vi "DrumSequence_Cont_Execute.vi"(4 "Set Next Step":bool, 6 "Pass_Through_Time":dbl=-1.0 format="%33.4f", 7 "External Ready":bool=TRUE, 8 "Cancel Time Sec":dbl, 9 "Step Times Sec":dbl[](array[numeric]), 10 "Cancel":bool, 11 "Initiate":bool) -> (0 "Error":bool, 1 "Ready":bool, 2 "Seq  Active":bool, 3 "Step Number State":T1=enum."Initialize", 5 "New Step":bool)   [LabVIEW 2019, in "Trajectory_Library.lvlib"]
doc: "Implements a simplified state machine similar to a mechanical / electrical drum sequencer. When the Drum Sequencer is \"Ready\" and the \"Initiate\" input becomes TRUE,, the drum sequences through its set of steps from 1 to N. After each Step is executed it is followed by a wait. During the wait the Step output indicates \"Do Nothing\". The number of Steps is determined by the number of elements in the \"Step Times\" input array. Once all the steps have been executed, the Drum Sequencer cycles bac to wait for another initiate. \n\nThere is a Cancel input that interrupts the sequence, executes the Cancel Step, performs the cancel wait, and then returns to wait for an Initiate action. \n\nIf any of the Step Times, or Cancel times are negative, or there more than 32 steps, or less than 1 step an error is signaled. The drum sequencer selects the error state and stays there.\n\nInputs:\n\nOutputs:"
uses:
  Trajectory_Library.lvlib
  Enum/DrumSequence_Step_Enum.ctl
  Enum/DrumSequence_State_Enum.ctl
  Util_GetTime_U32.vi
  Util_GetTime_U64.vi
  <vilib>/Utility/semaphor.llb/Obtain Semaphore Reference.vi
  Timer_Reset.vi
panel:
  # "Time to wait\nafter executing\nstep"
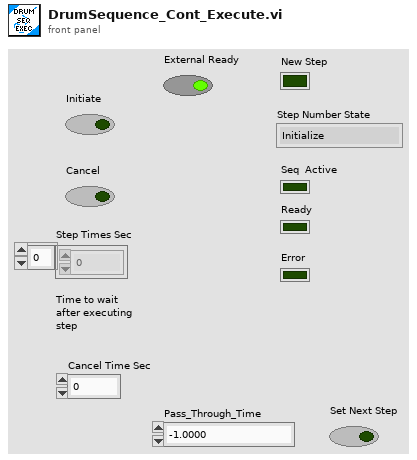
[diagram p1: front panel]
types:
  T1 = typedef "Trajectory_Library.lvlib/DrumSequence_Step_Enum.ctl" = enum16{"Do Nothing", "Step 1", "Step 2", "Step 3", "Step 4", "Step 5", "Step 6", "Step 7", "Step 8", "Step 9", "Step 10", "Step 11", "Step 12", "Step 13", "Step 14", "Step 15", "Step 16", "Step 17", "Step 18", "Step 19", "Step 20", "Step 21", "Step 22", "Step 23", "Step 24", "Step 25", "Step 26", "Step 27", "Step 28", "Step 29", "Step 30", "Step 31", "Step 32", "Cancel", "Initialize", "Error"}
  T2 = typedef "Trajectory_Library.lvlib/DrumSequence_State_Enum.ctl" = enum16{"Initialize", "Ready", "First Step", "Step Wait", "Next State", "Cancel", "Cancel Wait", "Error", "Error Loop"}
  T3 = typedef "Trajectory_Library.lvlib/TIMER.ctl" = cluster{"StartTime":dbl, "Accumulated TIme":dbl, "Running":bool, "semaphore":T4}
  T4 = typedef "Semaphore RefNum" = refnum<k1>
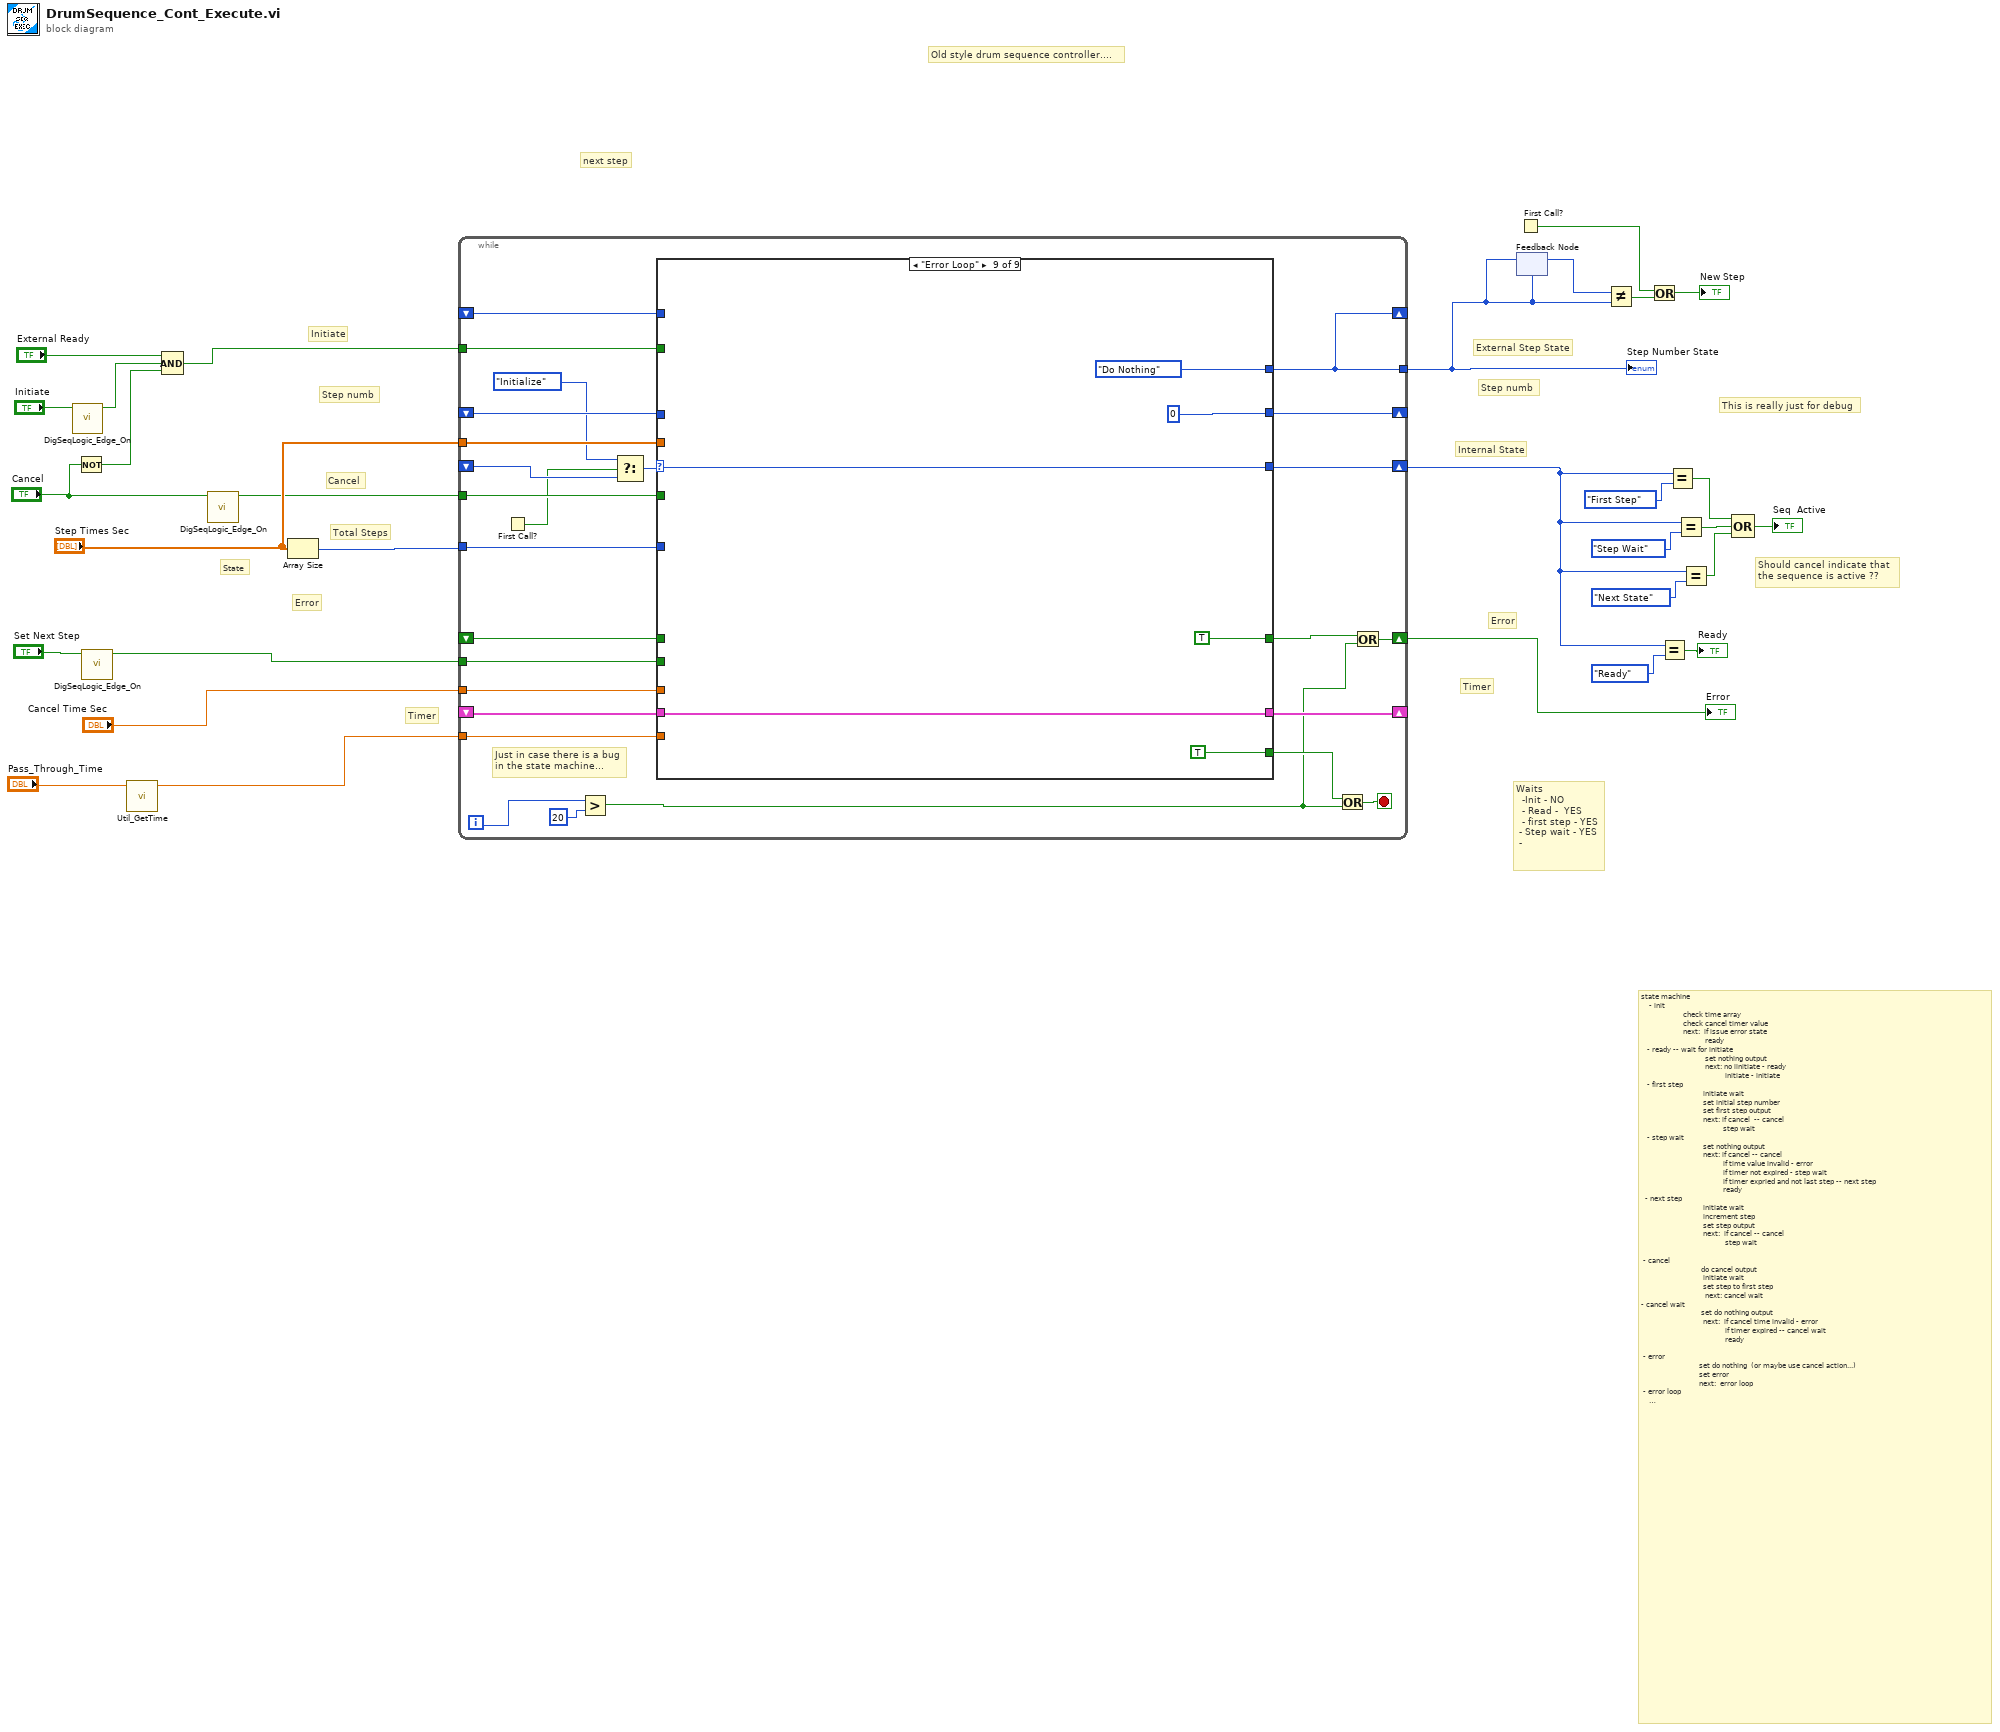
[diagram p0: block diagram]
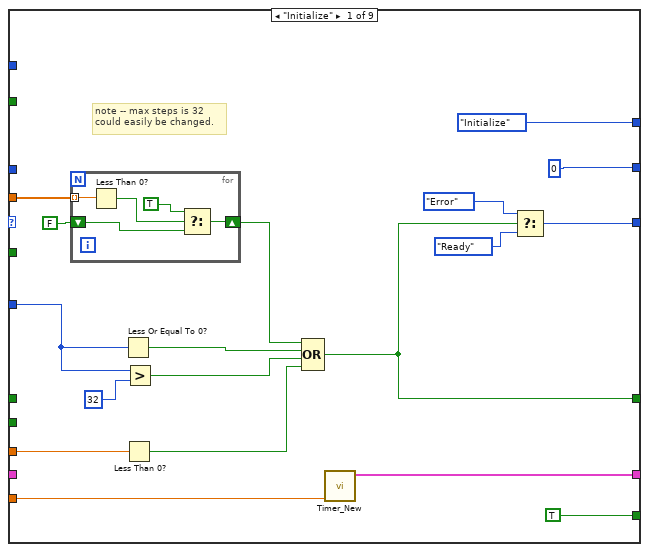
[diagram p2: hidden frame]
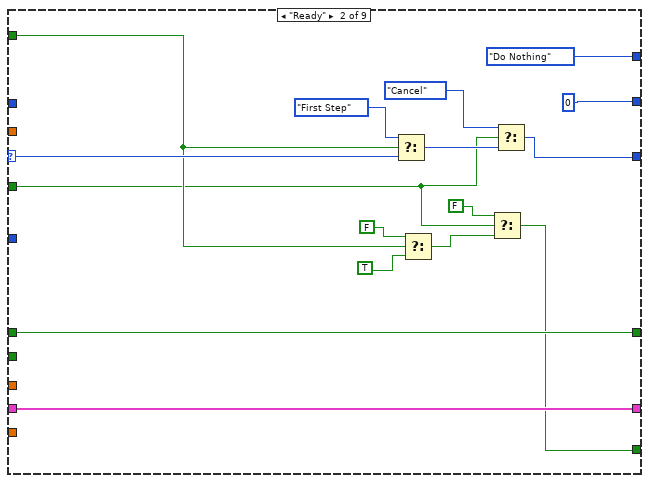
[diagram p3: hidden frame]
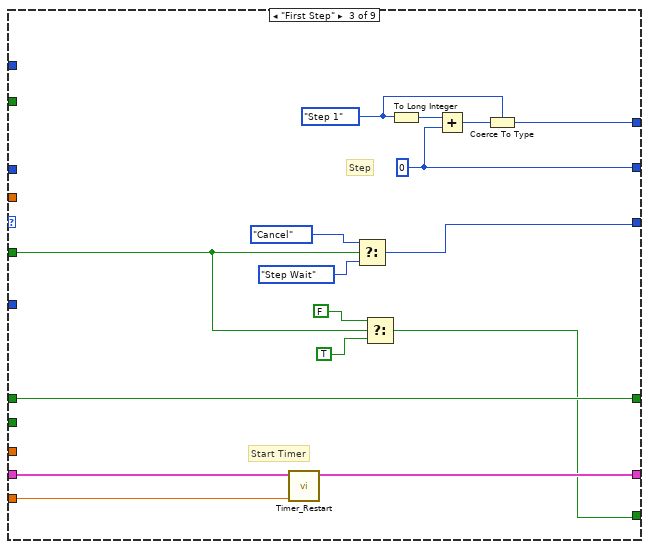
[diagram p4: hidden frame]
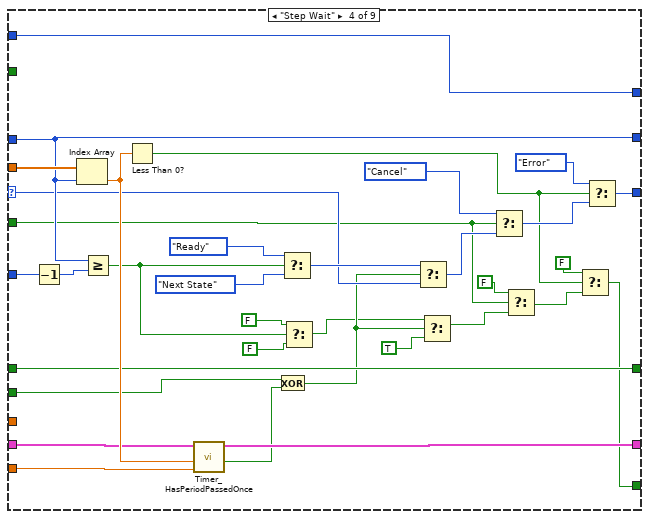
[diagram p5: hidden frame]
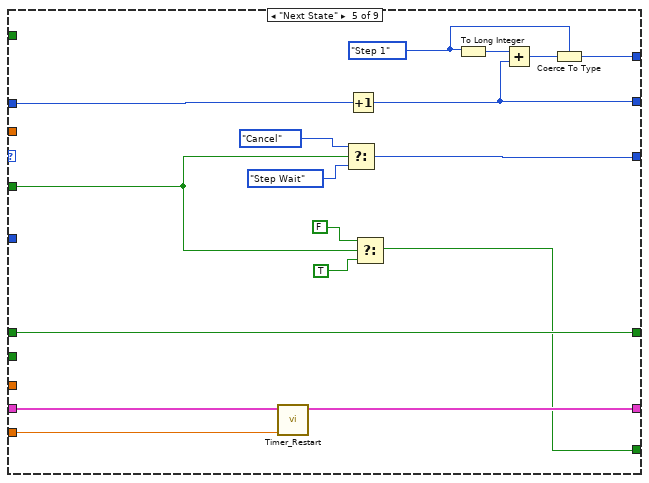
[diagram p6: hidden frame]
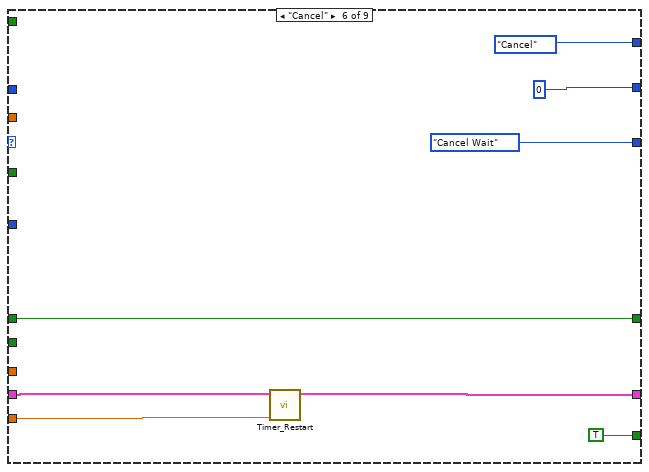
[diagram p7: hidden frame]
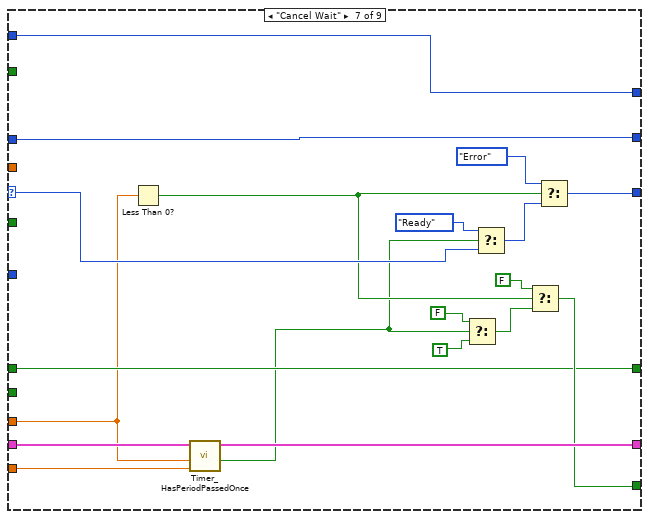
[diagram p8: hidden frame]
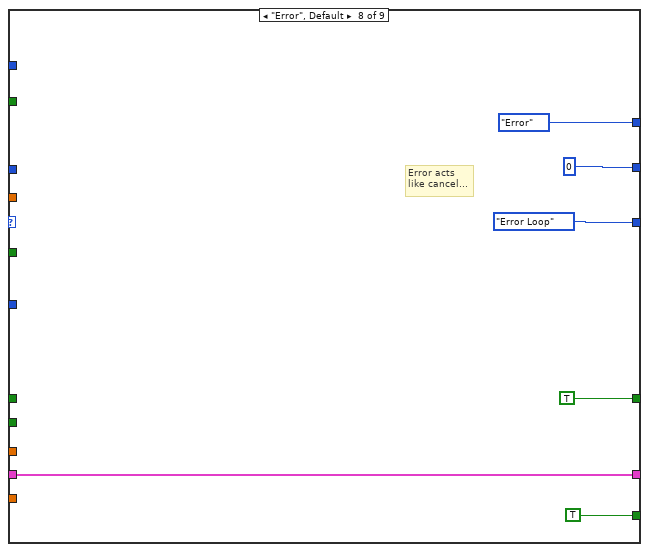
[diagram p9: hidden frame]
diagram:
  # "Should cancel indicate that\nthe sequence is active ??"
  # "This is really just for debug"
  # "Waits\n  -Init - NO\n  - Read -  YES\n  - first step - YES\n - Step wait - YES\n -"
  # "Timer"
  # "Error"
  # "State"
  # "Total Steps"
  # "Cancel"
  # "Step numb"
  # "Initiate"
  # "next step"
  # "Old style drum sequence controller...."
  # "Step numb"
  # "Timer"
  # "Error"
  # "Internal State"
  # "External Step State"
  # "state machine\n    - init\n                     check time array\n                     check cancel timer value\n                     next:  if issue error state\n                                ready\n   - ready -- wait for initiate\n                                set nothing output\n                                next: no iinitiate - ready\n                                          initiate - initiate\n   - first step \n                               initiate wait\n                               set initial step number\n                               set first step output\n                               next: if cancel  -- cancel\n                                         step wait\n   - step wait \n                               set nothing output\n                               next: if cancel -- cancel\n                                         if time value invalid - error\n                                         if timer not expired - step wait\n                                         if timer expried and not last step -- next step\n                                         ready\n  - next step\n                               initiate wait\n                               increment step\n                               set step output\n                               next:  if cancel -- cancel\n                                          step wait\n\n - cancel\n                              do cancel output\n                               initiate wait\n                               set step to first step\n                                next: cancel wait\n- cancel wait\n                              set do nothing output\n                               next:  if cancel time invalid - error\n                                          if timer expired -- cancel wait\n                                          ready\n\n - error\n                             set do nothing  (or maybe use cancel action...)\n                             set error\n                             next:  error loop\n - error loop\n                             set do nothing\n                             set error\n                             next: error loop"
  n1 = call "DigSeqLogic_Edge_On.vi"("Input"="Initiate") -> ("On Edge"=w28:bool)  [unwired: 10 in]
  n2 = Not(x="Cancel") -> (.not. x?=w30:bool)
  n3 = call "DigSeqLogic_Edge_On.vi"("Input"="Set Next Step") -> ("On Edge"=w9:bool)  [unwired: 10 in]
  n4 = call "Util_GetTime.vi"("Pass_Through_Time"="Pass_Through_Time") -> ("FPGA_Time_Seconds"=w23:dbl)  [unwired: 8 in, 2 out]
  n5 = Compound Arithmetic op=AND("External Ready", w28, w30) -> (w22:bool)
  n6 = call "DigSeqLogic_Edge_On.vi"("Input"="Cancel") -> ("On Edge"=w6:bool)  [unwired: 10 in]
  n7 = Array Size(array="Step Times Sec") -> (size(s)=w27:i32)
  n8 = while {
    tunnel: "Step Times Sec" -> [w55]
    tunnel: "Cancel Time Sec" -> [w54]
    tunnel: w23 -> [w53]
    tunnel: w22 -> [w52]
    tunnel: w6 -> [w51]
    tunnel: [w32] -> w1
    tunnel: w9 -> [w48]
    tunnel: w27 -> [w56]
    shift-right: [w47] -> _
    shift-left: _ -> [w41]
    shift-right: [w35] -> w8
    shift-left: _ -> [w46]
    shift-right: [w49] -> w12
    shift-left: _ -> [w43]
    shift-right: [w50] -> _
    shift-left: _ -> [w45]
    shift-right: [w32] -> _
    shift-left: _ -> [w31]
    i -> [w37]
    stop <- w39 stop-if-true
    # "Just in case there is a bug\nin the state machine..."
    n9 = First Call?() -> (First Call?: T/F=w40:bool)
    n10 = Greater?(x=w37, y=20) -> (0:w33:bool)
    n11 = Select(t=DrumSequence_State_Enum."Initialize", s=w40, f=w43) -> (s? t:f=w44:T2)
    n12 = case shown="\"Error Loop\"" w44 {
      selector: w44 -> [_ w94 _ w132 _ _ w183 _ w200]
      tunnel: w56 -> [w63 _ _ w130 _ _ _ _ _]
      tunnel: w55 -> [w73 _ _ w138 _ _ _ _ _]
      tunnel: w54 -> [w72 _ _ _ _ _ w173 _ _]
      tunnel: [w69 w91 w101 w126 w148 w165 w176 TRUE TRUE] -> w34
      tunnel: [w66 w84 w96 w135 w155 DrumSequence_State_Enum."Cancel Wait" w186 DrumSequence_State_Enum."Error Loop" w200] -> w49
      tunnel: [w65 w90 w106 w144 w153 w168 w187 w190 w197] -> w47
      tunnel: w53 -> [w64 _ w107 w145 w154 w169 w175 _ _]
      tunnel: [DrumSequence_Step_Enum."Initialize" ("Step Number") DrumSequence_Step_Enum."Do Nothing" ("Step Number") w109 w112 w156 DrumSequence_Step_Enum."Cancel" ("Step Number") w171 DrumSequence_Step_Enum."Error" ("Step Number") DrumSequence_Step_Enum."Do Nothing" ("Step Number")] -> w32
      tunnel: w52 -> [_ w89 _ _ _ _ _ _ _]
      tunnel: [0 0 w108 w133 w157 0 w184 0 0] -> w50
      tunnel: w51 -> [_ w81 w100 w118 w149 _ _ _ _]
      tunnel: w45 -> [_ _ _ w133 w158 _ w184 _ _]
      tunnel: w48 -> [_ _ _ w128 _ _ _ _ _]
      tunnel: w41 -> [_ w90 w102 w127 w147 w163 w174 w190 w197]
      tunnel: w46 -> [_ w91 w101 w126 w148 w165 w176 _ _]
      tunnel: [TRUE w80 w97 w113 w146 TRUE w178 TRUE TRUE] -> w38
      tunnel: w31 -> [_ _ _ w112 _ _ w171 _ _]
      frame "Initialize" {
        # "note -- max steps is 32\ncould easily be changed."
        n13 = for {
          shift-right: [w78] -> w71
          shift-left: FALSE -> [w77]
          tunnel: w73 -> [w79] mode=indexing
          n14 = Less Than 0?(x=w79) -> (x < 0?=w75:bool)
          n15 = Select(t=TRUE, s=w75, f=w77) -> (s? t:f=w78:bool)
        }
        n16 = Less Or Equal To 0?(x=w63) -> (x <= 0?=w70:bool)
        n17 = Less Than 0?(x=w72) -> (x < 0?=w57:bool)
        n18 = Greater?(x=w63, y=32) -> (0:w58:bool)
        n19 = Compound Arithmetic op=OR(w71, w70, w58, w57) -> (w69:bool)
        n20 = call "Timer_New.vi"("Pass_Through_Time"=w64) -> ("TIMER"=w65:T3)  [unwired: 10 in]
        n21 = Select(t=DrumSequence_State_Enum."Error", s=w69, f=DrumSequence_State_Enum."Ready") -> (s? t:f=w66:T2)
      }
      frame "Ready" {
        n22 = Select(t=DrumSequence_State_Enum."First Step", s=w89, f=w94) -> (s? t:f=w85:T2)
        n23 = Select(t=FALSE, s=w89, f=TRUE) -> (s? t:f=w82:bool)
        n24 = Select(t=FALSE, s=w81, f=w82) -> (s? t:f=w80:bool)
        n25 = Select(t=DrumSequence_State_Enum."Cancel", s=w81, f=w85) -> (s? t:f=w84:T2)
      }
      frame "First Step" {
        w103 = DrumSequence_Step_Enum."Step 1" ("Step Number")
        w108 = 0
        # "Start Timer"
        # "Step"
        n26 = call "Timer_Restart.vi"("Pass_Through_Time"=w107, "in Timer"=w102) -> ("out Timer"=w106:T3)  [unwired: 9 in]
        n27 = Select(t=DrumSequence_State_Enum."Cancel", s=w100, f=DrumSequence_State_Enum."Step Wait") -> (s? t:f=w96:T2)
        n28 = Select(t=FALSE, s=w100, f=TRUE) -> (s? t:f=w97:bool)
        n29 = To Long Integer(number=w103) -> (32bit integer=w111:i32)
        n30 = Add(x=w111, y=w108) -> (x+y=w110:i32)
        n31 = Coerce To Type(0:w110, 1:w103) -> (2:w109:T1)
      }
      frame "Step Wait" {
        n32 = Decrement(x=w130) -> (x-1=w131:i32)
        n33 = Index Array(array=w138, index=w133) -> (element=w137:dbl)
        n34 = Greater Or Equal?(x=w133, y=w131) -> (x >= y?=w125:bool)
        n35 = Less Than 0?(x=w137) -> (x < 0?=w114:bool)
        n36 = call "Timer_HasPeriodPassedOnce.vi"("Pass_Through_Time"=w145, "Period"=w137, "in Timer"=w127) -> ("Expired"=w129:bool, "out Timer"=w144:T3)  [unwired: 6 in, 1 out]
        n37 = Exclusive Or(1:w129, 2:w128) -> (0:w122:bool)
        n38 = Select(t=DrumSequence_State_Enum."Ready", s=w125, f=DrumSequence_State_Enum."Next State") -> (s? t:f=w139:T2)
        n39 = Select(t=FALSE, s=w125, f=FALSE) -> (s? t:f=w121:bool)
        n40 = Select(t=w139, s=w122, f=w132) -> (s? t:f=w142:T2)
        n41 = Select(t=w121, s=w122, f=TRUE) -> (s? t:f=w119:bool)
        n42 = Select(t=DrumSequence_State_Enum."Cancel", s=w118, f=w142) -> (s? t:f=w134:T2)
        n43 = Select(t=FALSE, s=w118, f=w119) -> (s? t:f=w115:bool)
        n44 = Select(t=FALSE, s=w114, f=w115) -> (s? t:f=w113:bool)
        n45 = Select(t=DrumSequence_State_Enum."Error", s=w114, f=w134) -> (s? t:f=w135:T2)
      }
      frame "Next State" {
        w152 = DrumSequence_Step_Enum."Step 1" ("Step Number")
        n46 = call "Timer_Restart.vi"("Pass_Through_Time"=w154, "in Timer"=w147) -> ("out Timer"=w153:T3)  [unwired: 9 in]
        n47 = Select(t=DrumSequence_State_Enum."Cancel", s=w149, f=DrumSequence_State_Enum."Step Wait") -> (s? t:f=w155:T2)
        n48 = Increment(x=w158) -> (x+1=w157:i32)
        n49 = Select(t=FALSE, s=w149, f=TRUE) -> (s? t:f=w146:bool)
        n50 = To Long Integer(number=w152) -> (32bit integer=w162:i32)
        n51 = Add(x=w162, y=w157) -> (x+y=w161:i32)
        n52 = Coerce To Type(0:w161, 1:w152) -> (2:w156:T1)
      }
      frame "Cancel" {
        n53 = call "Timer_Restart.vi"("Pass_Through_Time"=w169, "in Timer"=w163) -> ("out Timer"=w168:T3)  [unwired: 9 in]
      }
      frame "Cancel Wait" {
        n54 = Less Than 0?(x=w173) -> (x < 0?=w177:bool)
        n55 = call "Timer_HasPeriodPassedOnce.vi"("Pass_Through_Time"=w175, "Period"=w173, "in Timer"=w174) -> ("Expired"=w172:bool, "out Timer"=w187:T3)  [unwired: 6 in, 1 out]
        n56 = Select(t=FALSE, s=w172, f=TRUE) -> (s? t:f=w182:bool)
        n57 = Select(t=DrumSequence_State_Enum."Ready", s=w172, f=w183) -> (s? t:f=w188:T2)
        n58 = Select(t=FALSE, s=w177, f=w182) -> (s? t:f=w178:bool)
        n59 = Select(t=DrumSequence_State_Enum."Error", s=w177, f=w188) -> (s? t:f=w186:T2)
      }
      frame "Error", Default {
        # "Error acts\nlike cancel..."
      }
      frame "Error Loop" {
      }
    }
    n60 = Or(x=w38, y=w33) -> (x .or. y?=w39:bool)
    n61 = Or(x=w34, y=w33) -> (x .or. y?=w35:bool)
  }
  "Error" <- w8
  "Step Number State" <- w1
  n62 = First Call?() -> (First Call?: T/F=w2:bool)
  n63 = feedback #1(w1) -> (w5:T1)
  n64 = feedback-in #1(w1) -> ()
  n65 = Not Equal?(x=w5, y=w1) -> (x != y?=w3:bool)
  n66 = Or(x=w2, y=w3) -> (x .or. y?=→"New Step":bool)
  n67 = Equal?(x=w12, y=DrumSequence_State_Enum."Ready") -> (x = y?=→"Ready":bool)
  n68 = Equal?(x=w12, y=DrumSequence_State_Enum."First Step") -> (x = y?=w16:bool)
  n69 = Equal?(x=w12, y=DrumSequence_State_Enum."Step Wait") -> (x = y?=w15:bool)
  n70 = Equal?(x=w12, y=DrumSequence_State_Enum."Next State") -> (x = y?=w14:bool)
  n71 = Compound Arithmetic op=OR(w16, w15, w14) -> (→"Seq  Active":bool)
